vi "getZThXThYbow.vi"(10 "PosMeas_ZeroOffset":fxp<+/-,25,5>[](array[numeric])=[0.0, 0.0, 0.0, 0.0, 0.0], 11 "PosMeas_Array In":fxp<+/-,25,5>[](array[numeric])=[0.0, 0.0, 0.0, 0.0, 0.0, 0.0, 0.0, 0.0, 0.0, 0.0, 0.0, 0.0, 0.0]) -> (3 "Z,ThX,ThY,Bow_out":fxp<+/-,25,5>[](array[numeric]))   [LabVIEW 2020, in "PositionMeas.lvlib"]
doc: "Returns the Z, ThX, ThY, and Bow measurements based on position sensor data"
uses:
  PositionMeas.lvlib
  <vilib>/Platform/TimedLoop/XDataNode/XDataNode.xnode
  <vilib>/Platform/TimedLoop/XDataNode/nitl_modes.ctl
  <vilib>/Platform/TimedLoop/XDataNode/XDNodeRunTimeDep.lvlib
  <vilib>/Platform/TimedLoop/XDataNode/wakeup.ctl
  <vilib>/Platform/TimedLoop/XDataNode/timing_clust.ctl
  <vilib>/rvi/FXPMathLib/FxpSub/XNode/nifxpmath_Sub.xnode
  <vilib>/rvi/FXPMathLib/sim/FxpSim.dll
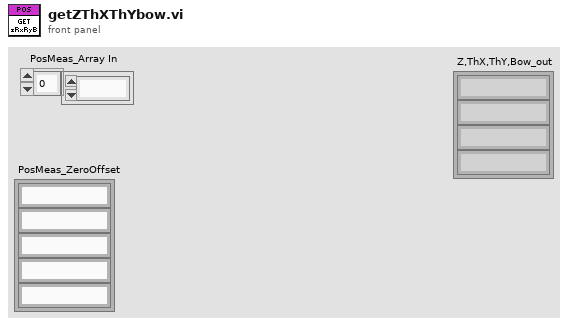
[diagram p1: front panel]
types:
  T1 = typedef "XDNodeRunTimeDep.lvlib/timing_clust.ctl" = cluster{"Expected End [f-1]":u64, "Actual End [f-1]":u64, "Finished Late? [f-1]":bool, "Expected End [i-1]":u64, "Actual End [i-1]":u64, "Finished Late? [i-1]":bool, "Expected Start [i]":u64, "Actual Start [i]":u64, "Expected Start [f]":u64, "Actual Start [f]":u64, "Source Name":string, "Structure Name":string, "Period":i64, "Deadline":i64, "Offset":i64, "Start":i64, "Priority":i32, "Timeout":i32, "Mode":T2, "Wakeup Reason":T3, "Error":errorcluster, "Source Type":string, "Secondary Source Type":string, "Global End Time":u64, "Global Start Time":u64, "Frame Duration":u64, "Iteration Duration":u64, "Assigned CPU":i32, "I/O Scan Engine Mode":u32}
  T2 = typedef "XDNodeRunTimeDep.lvlib/nitl_modes.ctl" = enum32{"No Change", "Process missed periods, maintain original phase", "Discard missed periods, maintain original phase", "Process missed periods, ignore original phase", "Discard missed periods, ignore original phase"}
  T3 = typedef "XDNodeRunTimeDep.lvlib/wakeup.ctl" = enum32{"Normal", "Aborted", "Asynchronous wakeup", "Timing source error", "Timed loop error", "Timeout"}
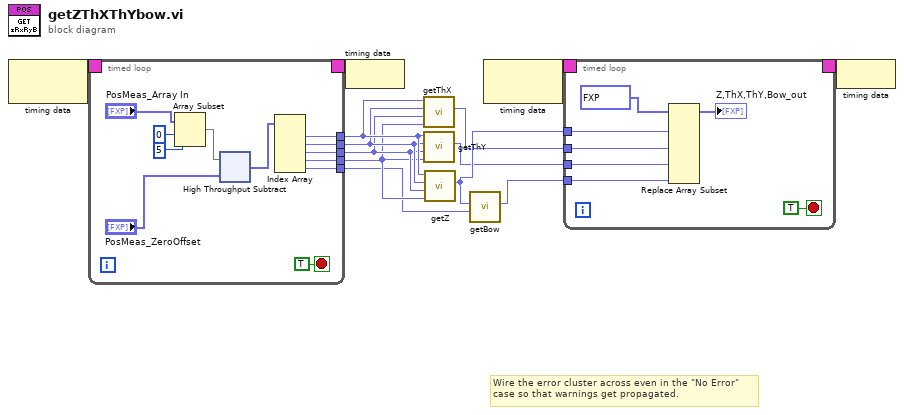
[diagram p0: block diagram]
diagram:
  # "Wire the error cluster across even in the \"No Error\"\ncase so that warnings get propagated."
  n1 = node-c288() -> (w2:T1)  [unwired: 1 in]
  n2 = timed-loop {
    timing: w2 -> [_]
    timing-out: [_] -> w1
    tunnel: [w25] -> w11
    tunnel: [w24] -> w10
    tunnel: [w23] -> w9
    tunnel: [w22] -> w8
    tunnel: [w21] -> w7
    stop <- TRUE stop-if-true
    n3 = Array Subset(array="PosMeas_Array In", index=0, length=5) -> (w16:fxp<+/-,25,5>[])
    n4 = xnode ("High Throughput Subtract")("x"=w16, "y"="PosMeas_ZeroOffset") -> ("x-y"=w14:fxp<+/-,25,5>[])
    n5 = Index Array(array=w14) -> (element #1=w25:fxp<+/-,25,5>, element #2=w24:fxp<+/-,25,5>, element #3=w23:fxp<+/-,25,5>, element #4=w22:fxp<+/-,25,5>, element #5=w21:fxp<+/-,25,5>)  [unwired: 5 in]
  }
  n6 = node-c288(w1) -> ()
  n7 = call "getThX.vi"("SW"=w8, "NW"=w9, "NE"=w10, "SE"=w11) -> ("ThX"=w5:fxp<+/-,25,5>)  [unwired: 7 in]
  n8 = call "getThY.vi"("SW"=w8, "NW"=w9, "NE"=w10, "SE"=w11) -> ("ThY"=w4:fxp<+/-,25,5>)  [unwired: 7 in]
  n9 = call "getZ.vi"("SW"=w8, "NW"=w9, "NE"=w10, "SE"=w11) -> ("Z"=w6:fxp<+/-,25,5>)  [unwired: 7 in]
  n10 = call "getBow.vi"("CI"=w7, "Z"=w6) -> ("Bow"=w3:fxp<+/-,25,5>)  [unwired: 9 in]
  n11 = node-c288() -> (w13:T1)  [unwired: 1 in]
  n12 = timed-loop {
    timing: w13 -> [_]
    timing-out: [_] -> w12
    tunnel: w6 -> [w34]
    tunnel: w5 -> [w33]
    tunnel: w4 -> [w32]
    tunnel: w3 -> [w31]
    stop <- TRUE stop-if-true
    n13 = Replace Array Subset(array=fxp<+/-,25,5>[] [0.0, 0.0, 0.0, 0.0], new element #1=w34, new element #2=w33, new element #3=w32, new element #4=w31) -> (→"Z,ThX,ThY,Bow_out":fxp<+/-,25,5>[])  [unwired: 4 in]
  }
  n14 = node-c288(w12) -> ()
